vi "Fwd Kin.vi"(11 "Joint Coordinates (rad)":dbl[](array[numeric])) -> (0 "E_theta (deg)":dbl, 3 "Task Coordinates (cm)":dbl[](array[numeric]))   [LabVIEW 2019]
panel:
  # "Theta 0"
  # "Ex"
  # "Ey"
  # "Theta 1"
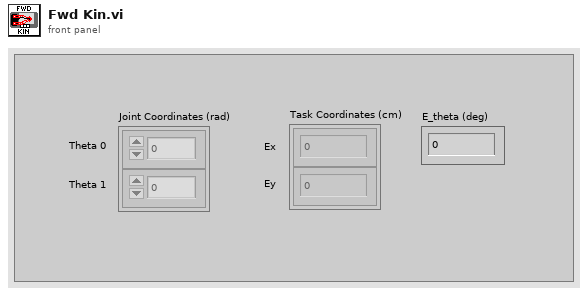
[diagram p1: front panel]
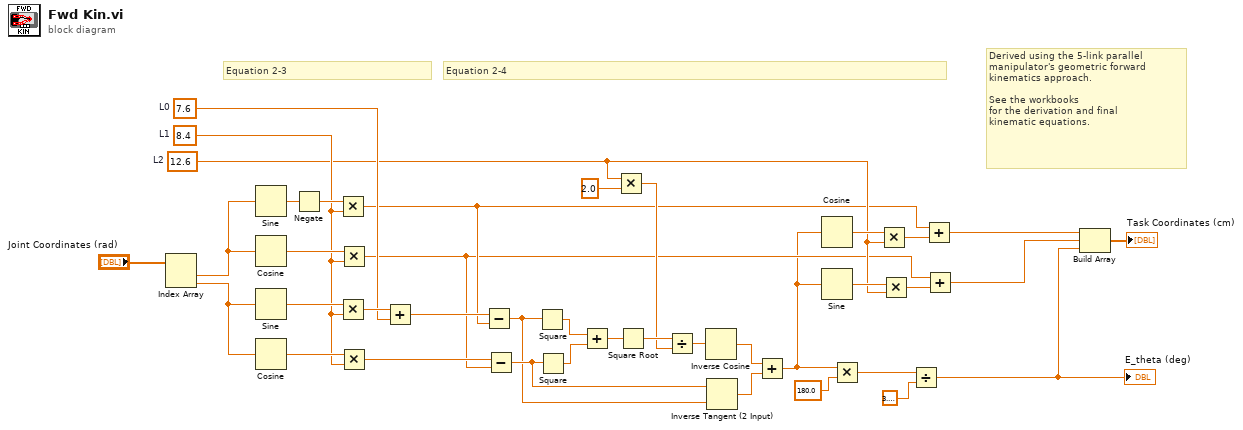
[diagram p0: block diagram]
diagram:
  w16 = 12.6  # L2
  w34 = 8.4  # L1
  w32 = 7.6  # L0
  # "Derived using the 5-link parallel \nmanipulator's geometric forward \nkinematics approach. \n\nSee the workbooks\nfor the derivation and final\nkinematic equations."
  # "Equation 2-4"
  # "Equation 2-3"
  n1 = Index Array(array="Joint Coordinates (rad)") -> (element #1=w6:dbl, element #2=w5:dbl)  [unwired: 2 in]
  n2 = Sine(x=w6) -> (sin(x)=w37:dbl)
  n3 = Cosine(x=w6) -> (cos(x)=w39:dbl)
  n4 = Sine(x=w5) -> (sin(x)=w35:dbl)
  n5 = Cosine(x=w5) -> (cos(x)=w36:dbl)
  n6 = Negate(x=w37) -> (-x=w38:dbl)
  n7 = Multiply(x=w38, y=w34) -> (x*y=w14:dbl)
  n8 = Multiply(x=w35, y=w34) -> (x*y=w33:dbl)
  n9 = Multiply(x=w39, y=w34) -> (x*y=w12:dbl)
  n10 = Multiply(x=w36, y=w34) -> (x*y=w30:dbl)
  n11 = Add(x=w33, y=w32) -> (x+y=w31:dbl)
  n12 = Subtract(x=w31, y=w14) -> (x-y=w28:dbl)
  n13 = Subtract(x=w30, y=w12) -> (x-y=w29:dbl)
  n14 = Square(x=w28) -> (x^2=w27:dbl)
  n15 = Square(x=w29) -> (x^2=w26:dbl)
  n16 = Add(x=w27, y=w26) -> (x+y=w25:dbl)
  n17 = Multiply(x=w16, y=2.0) -> (x*y=w22:dbl)
  n18 = Square Root(x=w25) -> (sqrt(x)=w23:dbl)
  n19 = Divide(x=w23, y=w22) -> (x/y=w21:dbl)
  n20 = Inverse Cosine(1:w21) -> (0:w20:dbl)
  n21 = Inverse Tangent (2 Input)(1:w28, 2:w29) -> (0:w19:dbl)
  n22 = Add(x=w20, y=w19) -> (x+y=w11:dbl)
  n23 = Cosine(x=w11) -> (cos(x)=w18:dbl)
  n24 = Sine(x=w11) -> (sin(x)=w17:dbl)
  n25 = Multiply(x=w11, y=180.0) -> (x*y=w9:dbl)
  n26 = Multiply(x=w18, y=w16) -> (x*y=w15:dbl)
  n27 = Multiply(x=w17, y=w16) -> (x*y=w13:dbl)
  n28 = Divide(x=w9, y=3.141592653589793) -> (x/y=w1:dbl)
  "E_theta (deg)" <- w1
  n29 = Add(x=w14, y=w15) -> (x+y=w4:dbl)
  n30 = Add(x=w12, y=w13) -> (x+y=w3:dbl)
  n31 = Build Array(w4, w3, w1) -> (→"Task Coordinates (cm)":dbl[])
